vi "Move YZ Raster + C-Scan.vi"(0 "Reference In":refnum<class "_Controller.lvclass">, 1 "Y Number of Steps":string="0", 2 "VISA resource name":refnum<visa-resource-name>, 3 "Source (0: Channel 1)":u16(ring) items=["Channel 1", "Channel 2", "Channel 3", "Channel 4", "Memory 1", "Memory 2", "Memory 3", "Memory 4", "Function 1", "Function 2", "Function 3", "Function 4", "Function 5", "Function 6", "Function 7", "Function 8"], 4 "Z Number of Steps":string="0", 5 "Error In":errorcluster, 8 "C-Scan Build Up Quantity":T1(radio), 9 "Initial Y Direction":bool=TRUE, 11 "Initial Z Direction":bool=TRUE) -> (14 "Reference Out":refnum<class "_Controller.lvclass">, 15 "A-Scan (for C-Scan)":waveform(dbl)[](graph), 16 "C-Scan":dbl[][](array[numeric]), 19 "Error Out":errorcluster)   [LabVIEW 2020]
doc: "Bi-axial raster scan logic for the YZ plane inclduing the processing to obtain a C-scan from all the indiviual A-scans. Performs the uni-axial raster scan logic in the Y direction then moves along 1 scanning point in the Z dirction. This is the looped to cover the entire area.\n\nArgs:\n\nReference In: Incoming communication (reference) between LabView and the scanning rig controller\nY Number of Steps: Total number of steps to move along that axis\nZ Number of Steps: Total number of steps to move along that axis\nInitial Y Direction: Initial Y direction for the scan\nInitial Z Direction: Initial Z direction for the scan\nC-Scan Build Up Quantity: Specifies the quantity used to build up the C-Scan image\nVISA Resource Name: Specifies the model of osciloscope being used\nSource (Channel): Specifies the channel to trigger for a reading on the osciloscope\nError In: Checks for any errors with the incoming communication (reference)\n\nReturns:\n\nReference Out: Output communnication (reference) between LabView and controller\nError Out: Checks for any error with output communication (reference)\nC-Scan: Output C-scan\nA-Scan: All the A-scan's taken for the entire plane"
uses:
  <instrlib>/Arcus Ethernet Driver 1.0.0/ArcusEthernetComm/classes/Controller/_Controller.lvclass
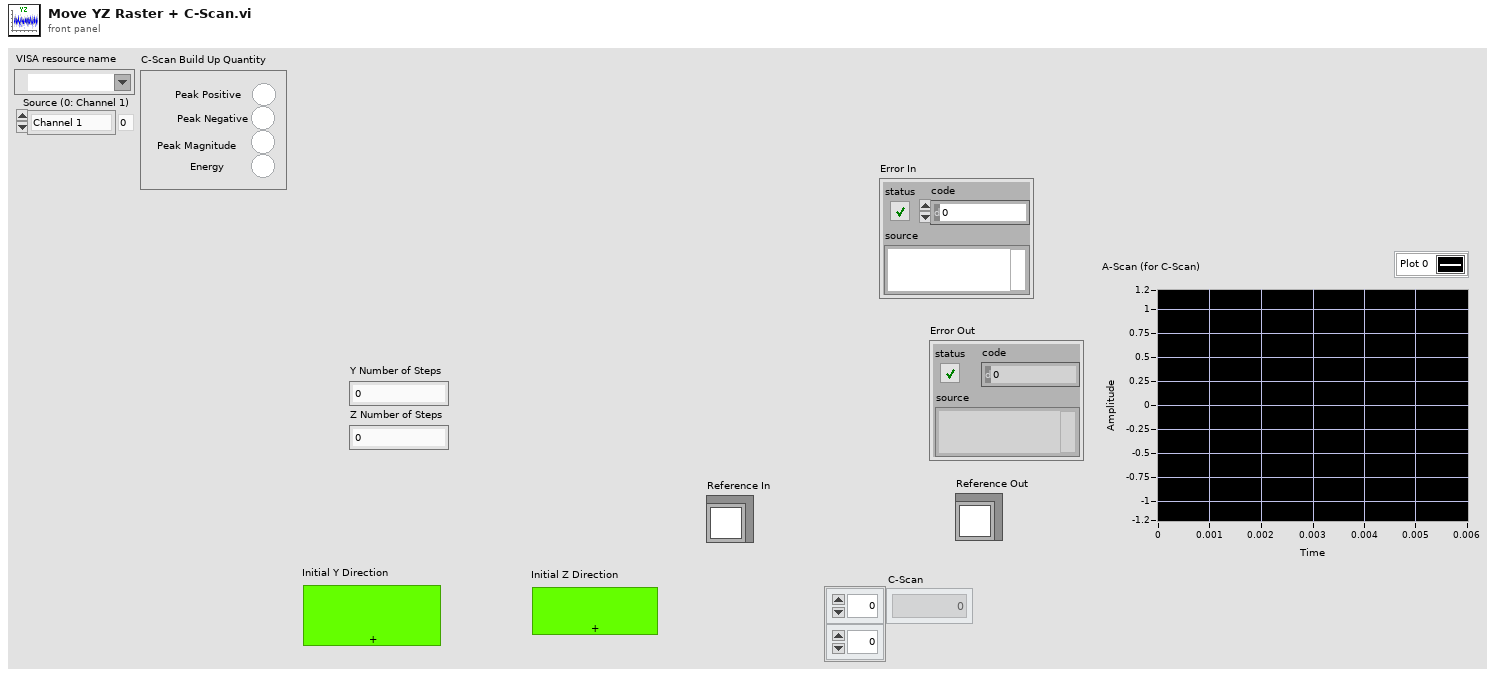
[diagram p1: front panel]
types:
  T1 = enum32{"No Selection", "Peak Positive", "Peak Negative", "Peak Magnitude", "Energy"}
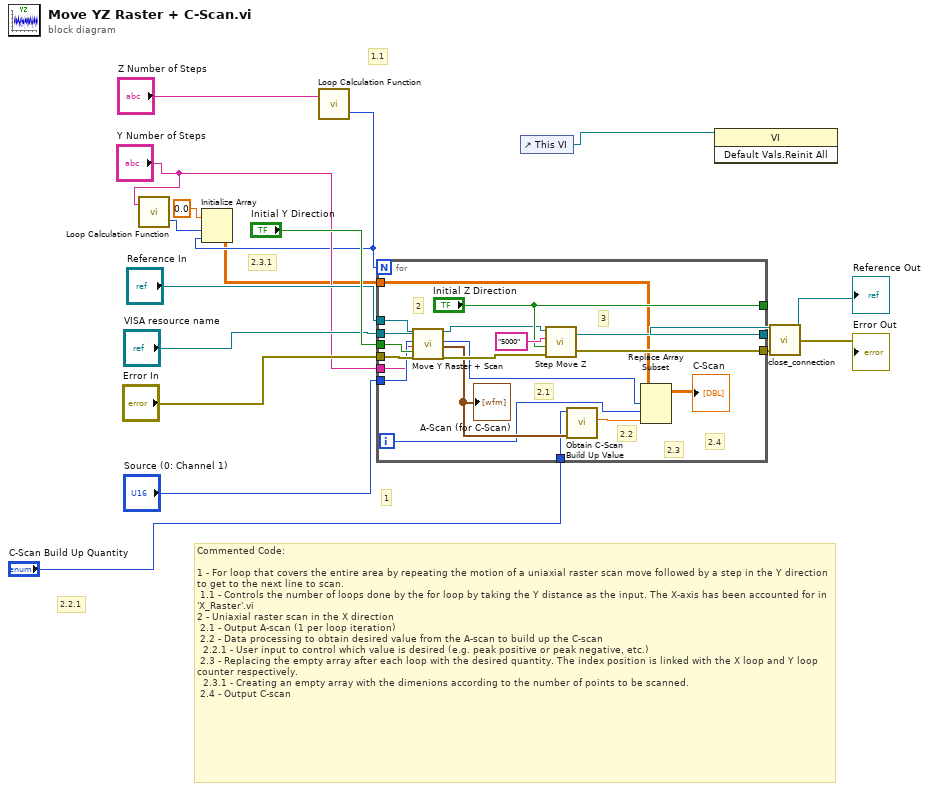
[diagram p0: block diagram]
diagram:
  # "2.2.1"
  # "2.3.1"
  # "Commented Code:\n\n1 - For loop that covers the entire area by repeating the motion of a uniaxial raster scan move followed by a step in the Y direction to get to the next line to scan.  \n 1.1 - Controls the number of loops done by the for loop by taking the Y distance as the input. The X-axis has been accounted for in 'X_Raster'.vi\n2 - Uniaxial raster scan in the X direction\n 2.1 - Output A-scan (1 per loop iteration)\n 2.2 - Data processing to obtain desired value from the A-scan to build up the C-scan\n  2.2.1 - User input to control which value is desired (e.g. peak positive or peak negative, etc.)\n 2.3 - Replacing the empty array after each loop with the desired quantity. The index position is linked with the X loop and Y loop counter respectively. \n  2.3.1 - Creating an empty array with the dimenions according to the number of points to be scanned.\n 2.4 - Output C-scan"
  # "1.1"
  # "1"
  n1 = call "Loop Calculation Function.vi"("Number of Steps"="Y Number of Steps") -> ("No. of Scan Points"=w4:i32)  [unwired: 1 in, 1 out]
  n2 = call "Loop Calculation Function.vi"("Number of Steps"="Z Number of Steps") -> ("No. of Scan Points"=w3:i32)  [unwired: 1 in, 1 out]
  n3 = Initialize Array(0.0 ("element"), w4, w3) -> (w1:dbl[][])
  n4 = for {
    N: w3 -> [_]
    tunnel: "Initial Y Direction" -> [w35]
    tunnel: ["Initial Z Direction"] -> _
    tunnel: [w32] -> w10
    tunnel: [w31] -> w9
    tunnel: "Reference In" -> [w29]
    tunnel: "Error In" -> [w28]
    tunnel: "VISA resource name" -> [w27]
    tunnel: "Source (0: Channel 1)" -> [w26]
    tunnel: "Y Number of Steps" -> [w25]
    tunnel: "C-Scan Build Up Quantity" -> [w21]
    tunnel: w1 -> [w18]
    i -> [w20]
    # "3"
    # "2.3"
    # "2.4"
    # "2.2"
    # "2.1"
    # "2"
    n5 = call "Move Y Raster + Scan.vi"("Reference In"=w29, "VISA resource name"=w27, "Source (0: Channel 1)"=w26, "Y Number of Steps"=w25, "Initial Direction"=w35, "Error In"=w28) -> ("Reference Out"=w33:refnum<class "_Controller.lvclass">, "For Loop Counter"=w19:i32, "A-Scan"=w22:waveform(dbl)[], "Error Out"=w30:errorcluster)  [unwired: 10 in]
    "A-Scan (for C-Scan)" <- w22
    n6 = call "Step Move Z.vi"("Error In"=w30, "Direction"="Initial Z Direction", "No. of Z Steps"="5000" ("Y Steps"), "Reference In"=w33) -> ("Error Out"=w31:errorcluster, "Reference Out"=w32:refnum<class "_Controller.lvclass">)
    n7 = call "Obtain C-Scan Build Up Value.vi"("A-Scans"=w22, "C-Scan Build Up Quantity"=w21) -> ("Desired Value for C-Scan"=w24:dbl)  [unwired: 9 in]
    n8 = Replace Array Subset(array=w18, new element=w24, index (row)=w19, index (col)=w20) -> (→"C-Scan":dbl[][])
  }
  n9 = control-ref of="This VI"() -> (w12:refnum<vi>)
  n10 = invoke class="VI" method="Default Vals.Reinit All"(reference=w12) -> ()  [unwired: 2 in, 3 out]
  n11 = call <instrlib>:"close_connection.vi"("reference (in)"=w10, "error in (no error)"=w9) -> ("reference (out)"=→"Reference Out":refnum<class "_Controller.lvclass">, "error out"=→"Error Out":errorcluster)  [unwired: 16 in]
